vi "CreateDatabase.vi"(6 "delimiter":string=";", 8 "Error In":errorcluster, 9 "Database Availability":bool[](array[boolean]), 10 "Database path array":path[](array[path]), 11 "Selected Library URLs":string[](array[string])) -> (0 "Error Out":errorcluster)   [LabVIEW 2014]
doc: "<B>Copyright</B>: (c) MHWirth 2015.\n\nIf \"Database Availability\" is False, information of the shared variables for the relevant process is obtained, and saved in the CSV file whose path is provided. \n\nIf the type is not defined, Status will be \"Undefined Type\", and initialization stops at the shared variable index."
panel:
  out "Name - Type":string[][](array[string])
  out "Number of Deployed SV":i32
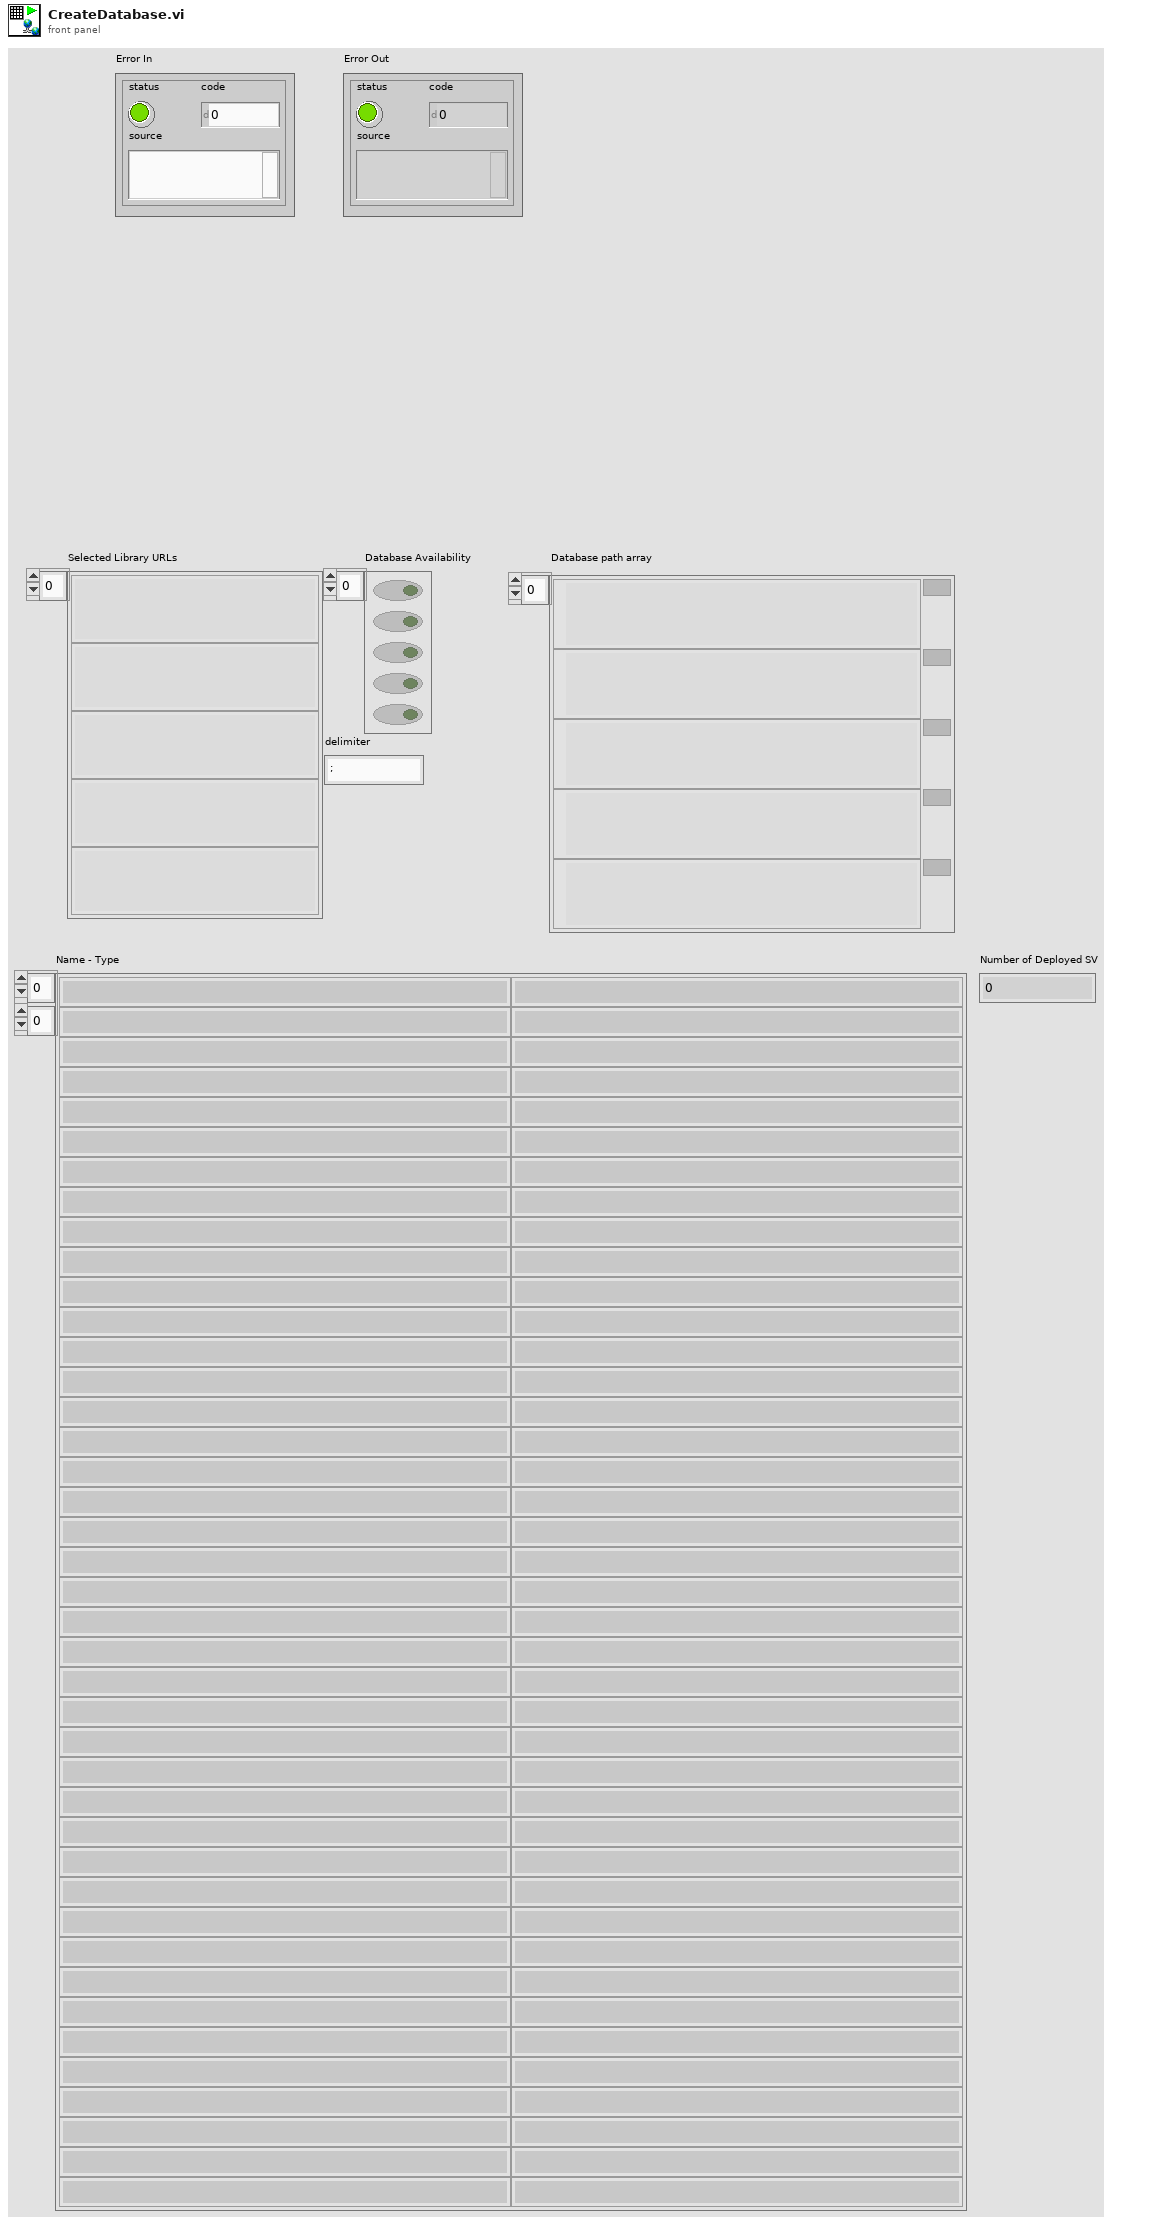
[diagram p1: front panel]
types:
  T1 = cluster{"Number of Variables":i32, "Variable/Parent Name array":string[][], "URL array":string[], "Type array":string[]}
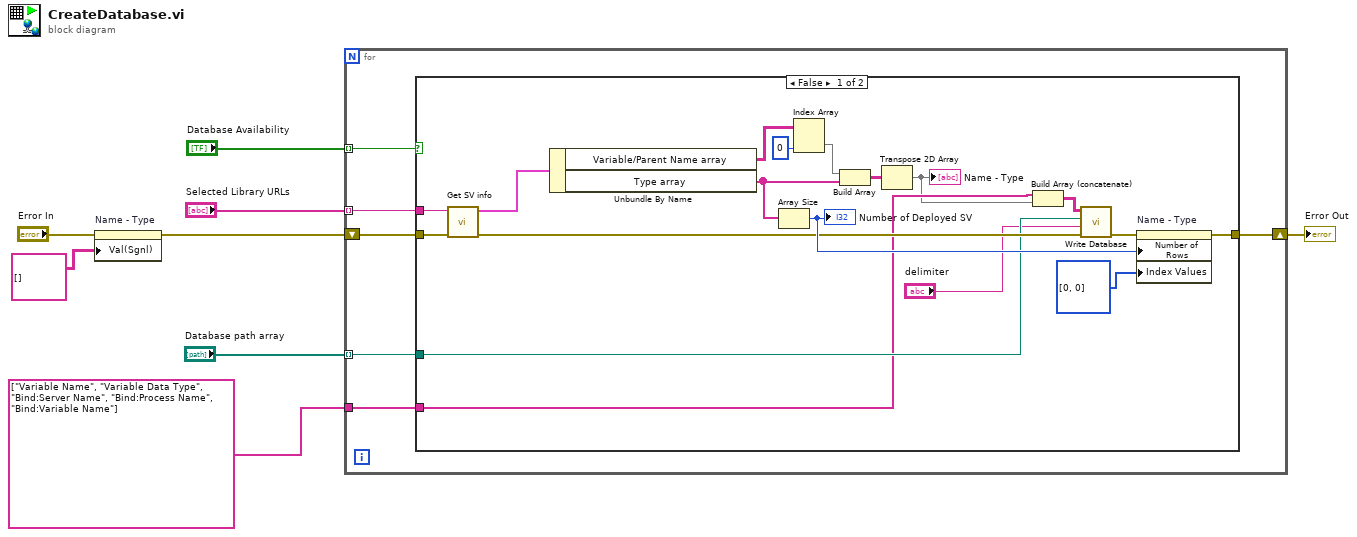
[diagram p0: block diagram]
diagram:
  n1 = property on="Name - Type" class="Arr (strict)"(error in="Error In", "Val(Sgnl)"=string[][] [] ("Value (Signaling)")) -> (error out=w2:errorcluster)  [unwired: 1 in, 1 out]
  n2 = for {
    shift-right: [w13] -> w3
    shift-left: w2 -> [w14]
    tunnel: "Database Availability" -> [w11] mode=indexing
    tunnel: "Database path array" -> [w10] mode=indexing
    tunnel: "Selected Library URLs" -> [w12] mode=indexing
    tunnel: string[] ["Variable Name", "Variable Data Type", "Bind:Server Name", "Bind:Process Name", "Bind:Variable Name"] -> [w9]
    n3 = case shown="False" w11 {
      tunnel: w14 -> [w32 w33]
      tunnel: [w24 w33] -> w13
      tunnel: w12 -> [w27 _]
      tunnel: w10 -> [w19 _]
      tunnel: w9 -> [w17 _]
      frame False {
        n4 = call "Get SV info.vi"("Error In"=w32, "container refnum in"=w27) -> ("Error Out"=w21:errorcluster, "Deployed Shared Variable Information"=w28:T1)  [unwired: 7 in, 1 out]
        n5 = Unbundle By Name(w28) -> ("Variable/Parent Name array"=w29:string[][], "Type array"=w25:string[])
        n6 = Array Size(array=w25) -> (size(s)=w23:i32)
        "Number of Deployed SV" <- w23
        n7 = Index Array(array=w29, index (col)=0 ("disabled index (col)")) -> (element=w26:string[])  [unwired: 1 in]
        n8 = Build Array(w26, w25) -> (w31:string[][])
        n9 = Transpose 2D Array(2D array=w31) -> (transposed array=w16:string[][])
        "Name - Type" <- w16
        n10 = Build Array (concatenate)(w17, w16) -> (w15:string[][])
        n11 = call "Write Database.vi"("Error In"=w21, "delimiter (\\t)"="delimiter", "DB Path"=w19, "Data in"=w15) -> ("Error Out"=w20:errorcluster)  [unwired: 7 in]
        n12 = property on="Name - Type" class="Arr (strict)"(error in=w20, "Number of Rows"=w23, "Index Values"=u32[] [0, 0] ("Selection Start[]")) -> (error out=w24:errorcluster)  [unwired: 1 in, 1 out]
      }
      frame True {
      }
    }
  }
  "Error Out" <- w3
